vi "ZK蠕动泵频率参数读取.vi"(7 "是否启用通讯通知":bool, 8 "error in (no error)":errorcluster, 11 "Slave ID":T1) -> (0 "error out":errorcluster, 2 "蠕动泵最小频率":i32, 3 "蠕动泵最大频率":i32)   [LabVIEW 2016, in "质控单元V4.lvlib"]
uses:
  <vilib>/Plasmionique/MB Master/MB_Master/MB_Master.lvclass
  <vilib>/Plasmionique/MB Master/MB Master.lvlib
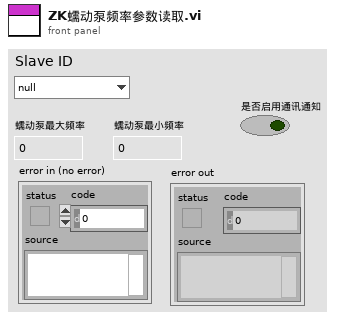
[diagram p1: front panel]
types:
  T1 = typedef "质控单元V4.lvlib/质控slave id.ctl" = enum16{"null", "氨氮", "总磷", "总氮", "CODMn", "CODCr"}
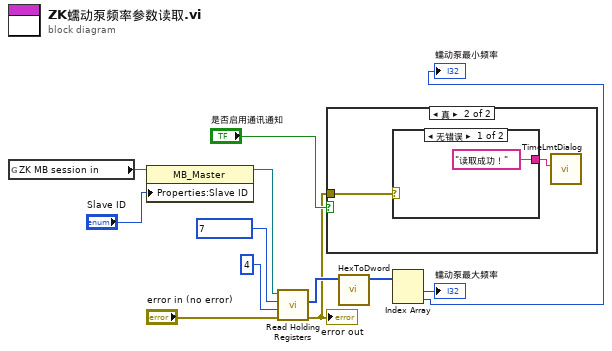
[diagram p0: block diagram]
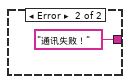
[diagram p3: hidden frame]
diagram:
  n1 = global read "ZK非断电保存全局变量.vi" "ZK MB session in"() -> (w11:refnum<class "MB_Master.lvclass">)
  n2 = property class="MB_Master"(reference=w11, "Properties:Slave ID"="Slave ID") -> (reference out=w9:refnum<class "MB_Master.lvclass">)  [unwired: 1 in, 1 out]
  n3 = call <vilib>:"Read Holding Registers.vi"("error in (no error)"="error in (no error)", "quantity"=u16 4, "starting address"=u16 7, "MB session in"=w9) -> ("error out"=w1:errorcluster, "Registers"=w6:u16[])  [unwired: 5 in, 1 out]
  "error out" <- w1
  n4 = case shown="真" "是否启用通讯通知" {
    tunnel: w1 -> [_ w14]
    frame False {
    }
    frame True {
      n5 = case shown="无错误" w14 {
        tunnel: ["读取成功！" "通讯失败！"] -> w13
        frame No Error {
        }
        frame Error {
        }
      }
      n6 = call "TimeLmtDialog.vi"("Infoin"=w13) -> ()  [unwired: 11 in]
    }
  }
  n7 = call "HexToDword.vi"("数组"=w6) -> ("DWORD"=w5:i32[])  [unwired: 10 in]
  n8 = Index Array(array=w5) -> (element #1=→"蠕动泵最大频率":i32, element #2=→"蠕动泵最小频率":i32)  [unwired: 2 in]
